vi "Dynamic Event Handler.vi"() -> ()   [LabVIEW 2021, in "Interaction Splitter.lvclass"]
doc: "Copyright 2018, Wiebe Walstra, wiebe@carya.nl."
uses:
  Interaction Splitter.lvclass
  Interaction Splitter.lvclass/Interaction Splitter.ctl
  <vilib>/event_ctls.llb/lveventtype.ctl
panel:
  in  "Interaction":refnum<class "Interaction Splitter.lvclass">
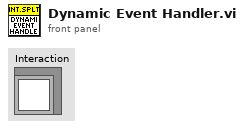
[diagram p1: front panel]
types:
  T1 = enum32{"Invalid", "Standard", "Closed", "Hidden", "Minimized", "Maximized"}
  T2 = enum32{"Bad", "Idle", "Run top level", "Running"}
  T3 = typedef "lveventtype.ctl" = enum32{"Null", "Timeout", "Annotation Menu Selection", "Annotation Menu Selection?", "App Instance Close", "App Instance Close?", "Autoscale Range Change", "Bookmark Info Change", "Cell Edit", "Cell Edit?", "Cursor Grab", "Cursor Grab?", "Cursor Menu Selection", "Cursor Menu Selection?", "Cursor Move", "Cursor Release", "Data Change", "Direction Change", "Display State Change", "Drag Ended", "Drag Enter", "Drag Leave", "Drag Over", "Drag Source Update", "Drag Starting", "Drag Starting?", "Drop", "Exec State Change", "Key Down", "Key Down?", "Key Repeat", "Key Repeat?", "Key Up", "Listbox Double Click", "Menu Activation?", "Menu Selection (App)", "Menu Selection? (App)", "Menu Selection (User)", "Mouse Down", "Mouse Down?", "Mouse Enter", "Mouse Leave", "Mouse Move", "Mouse Up", "Mouse Wheel", "NI Security User Change (App)", "Pane Size", "Panel Close", "Panel Close?", "Panel Resize", "Plot Attribute Change", "Scale Range Change", "Shortcut Menu Activation?", "Shortcut Menu Selection (App)", "Shortcut Menu Selection? (App)", "Shortcut Menu Selection (User)", "Tree Double Click", "Tree Drag", "Tree Drag?", "Tree Drop", "Tree Drop?", "Tree Item Close", "Tree Item Close?", "Tree Item Open", "Tree Item Open?", "User Event", "Value Change"}
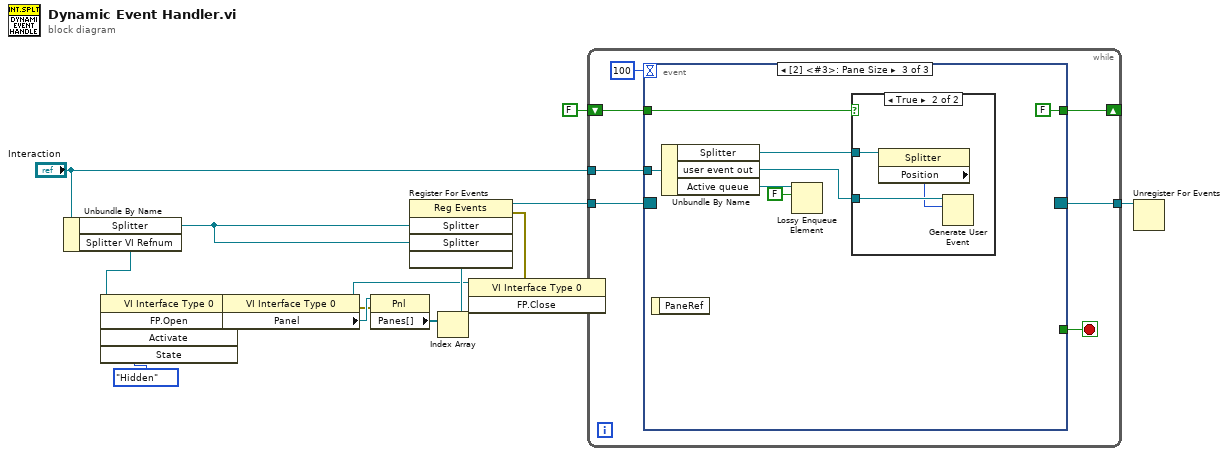
[diagram p0: block diagram]
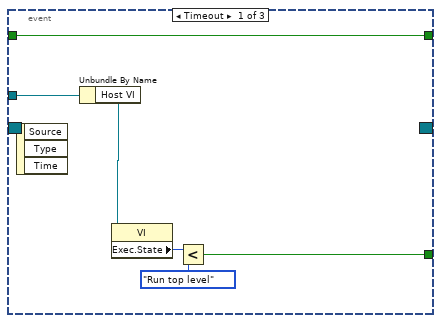
[diagram p2: hidden frame]
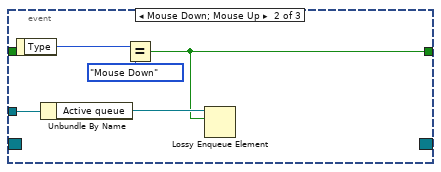
[diagram p3: hidden frame]
diagram:
  n1 = Unbundle By Name("Interaction") -> ("Splitter"=w13:refnum<vi>, "Splitter VI Refnum"=w6:refnum<vi>)
  n2 = invoke class="VI Interface Type 0" method="FP.Open"(reference=w6, "State"=T1."Hidden") -> (reference out=w5:refnum<vi>, error out=w2:errorcluster)  [unwired: 3 in, 3 out]
  n3 = property class="VI Interface Type 0"(reference=w5, error in=w2) -> (reference out=w4:refnum<vi>, error out=w10:errorcluster, "Panel"=w11:refnum<vi>)
  n4 = property class="Pnl"(reference=w11, error in=w10) -> ("Panes[]"=w12:refnum<vi>[])  [unwired: 2 out]
  n5 = Index Array(array=w12) -> (element=w9:refnum<vi>)  [unwired: 1 in]
  n6 = register-events(w13, w13, w9) -> (reference out=w15:refnum<event-registration>, error out=w3:errorcluster)  [unwired: 2 in]
  n7 = invoke class="VI Interface Type 0" method="FP.Close"(reference=w4, error in=w3) -> ()  [unwired: 1 in, 3 out]
  n8 = while {
    tunnel: w15 -> [w21]
    tunnel: "Interaction" -> [w20]
    shift-right: [w18] -> _
    shift-left: FALSE -> [w17]
    tunnel: [w16] -> w1
    stop <- w22 stop-if-true
    n9 = event shown="[2] <#3>: Pane Size" {
      selector: w21 -> [_ _ _]
      dyn-events: [_ _ _] -> w16
      timeout: 100 -> [_ _ _]
      tunnel: [w26 _ _] -> w22
      tunnel: w20 -> [w25 w31 w37]
      tunnel: [w23 w29 FALSE] -> w18
      tunnel: w17 -> [w23 _ w38]
      event Timeout {
        n10 = event-data() -> ()  [unwired: 1 in, 3 out]
        n11 = Unbundle By Name(w25) -> ("Host VI"=w24:refnum<vi>)
        n12 = property class="VI"(reference=w24) -> ("Exec.State"=w28:T2)  [unwired: 1 in, 2 out]
        n13 = Less?(x=w28, y=T2."Run top level" ("Execution:State")) -> (x < y?=w26:bool)
      }
      event Mouse Down; Mouse Up {
        n14 = event-data() -> ("Type"=w32:T3)  [unwired: 1 in]
        n15 = Unbundle By Name(w31) -> ("Active queue"=w30:refnum<queue>)
        n16 = Equal?(x=w32, y=lveventtype."Mouse Down" ("x")) -> (x = y?=w29:bool)
        n17 = Lossy Enqueue Element(queue=w30, element=w29) -> ()  [unwired: 1 in, 4 out]
      }
      event Pane Size {
        n18 = event-data() -> ()  [unwired: 1 in, 1 out]
        n19 = Unbundle By Name(w37) -> ("Splitter"=w39:refnum<vi>, "user event out"=w40:refnum<user-event>, "Active queue"=w34:refnum<queue>)
        n20 = Lossy Enqueue Element(queue=w34, element=FALSE) -> ()  [unwired: 1 in, 4 out]
        n21 = case shown="True" w38 {
          tunnel: w40 -> [_ w43]
          tunnel: w39 -> [_ w42]
          frame False {
          }
          frame True {
            n22 = property class="Splitter"(reference=w42) -> ("Position"=w41:i32)  [unwired: 1 in, 2 out]
            n23 = Generate User Event(user event=w43, event data cluster=w41) -> ()  [unwired: 2 in, 2 out]
          }
        }
      }
    }
  }
  n24 = Unregister For Events(event registration refnum=w1) -> ()  [unwired: 1 in, 1 out]
